vi "Init.vi"(5 "PathControl.lvclass":refnum<class "PathControl.lvclass">, 6 "Environmental classes":refnum<class "Instrument.lvclass">[](array[class]), 7 "XML Handler.lvclass":refnum<class "XML Handler.lvclass">, 8 "error in (no error)":errorcluster, 9 "Instruments to Use":T1(array[cluster]), 10 "Device.lvclass":refnum<class "Device.lvclass">, 11 "Power Meter GUI in":refnum<class "Power Meter GUI.lvclass">) -> (0 "error out":errorcluster, 3 "Power Meter GUI out":refnum<class "Power Meter GUI.lvclass">)   [LabVIEW 2020, in "Power Meter GUI.lvclass"]
doc: "Initializes the measurement.\nThis verifies that the instruments are present and adds them into the class data.\nIs also adds the xml handler into the class data."
uses:
  Power Meter GUI.lvclass
  C:/Sandbox/RF Bench/Source Code/WiSpry Test Framework/Measurements/Measurement.lvclass
  Devices/Device.lvclass
  Instruments/Instrument.lvclass
  XML Handler/XML Handler.lvclass
  Path Control/PathControl.lvclass
  Controls/Init State Machine.ctl
  Instruments/Power Meter/Power Meter.lvclass
  Measurement.lvclass/Measurement.ctl
  Measurement.lvclass
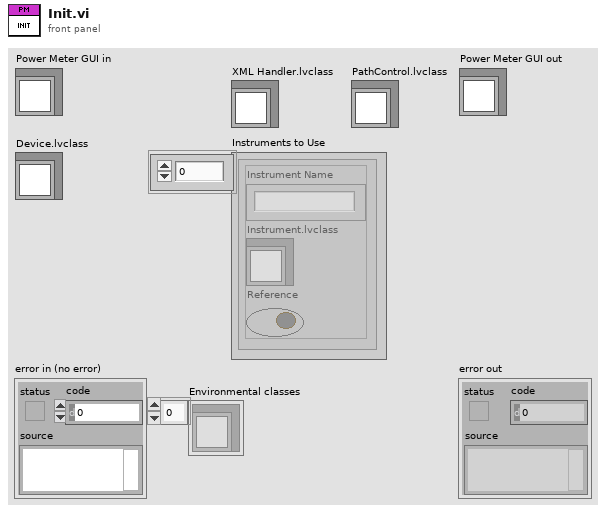
[diagram p1: front panel]
types:
  T1 = cluster{"Instrument Name":string, "Instrument.lvclass":refnum<class "Instrument.lvclass">, "Reference":bool}[]
  T2 = typedef "Power Meter GUI.lvclass/Init State Machine.ctl" = enum16{"Verify Instruments", "Init Instruments", "Init Device", "Create test in XML", "Set Path", "Done"}
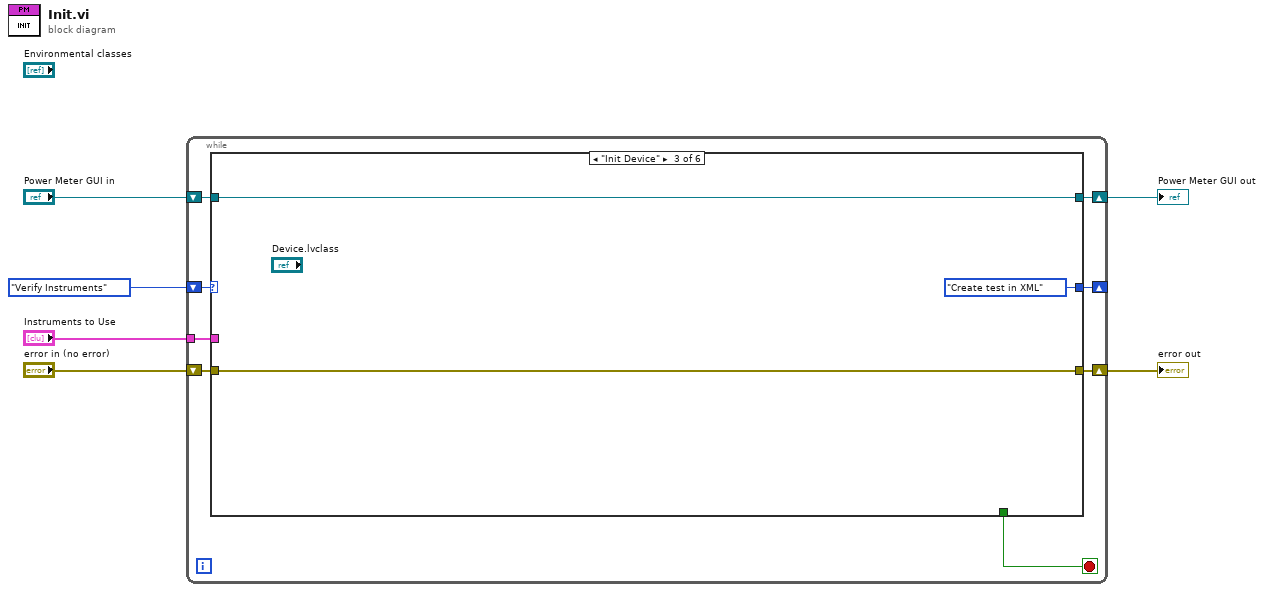
[diagram p0: block diagram]
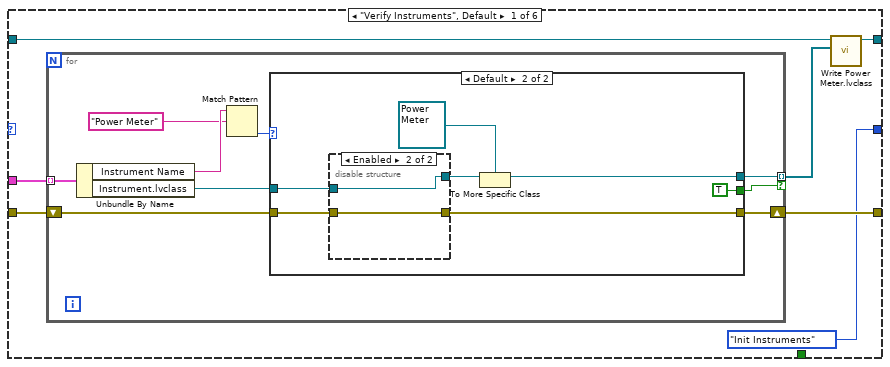
[diagram p2: hidden frame]
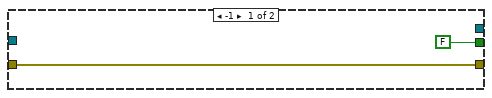
[diagram p3: hidden frame]
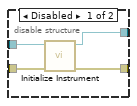
[diagram p4: hidden frame]
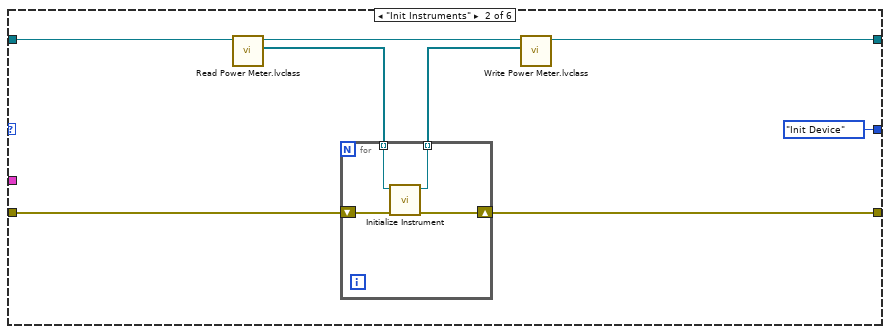
[diagram p5: hidden frame]
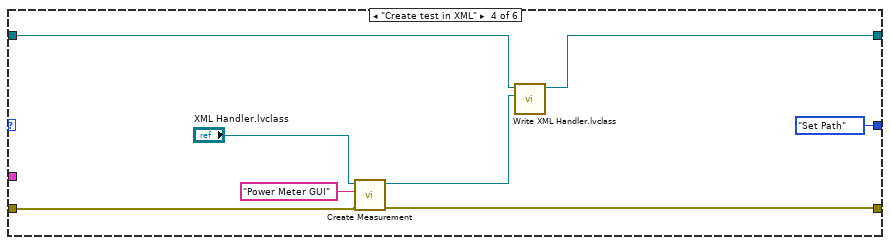
[diagram p6: hidden frame]
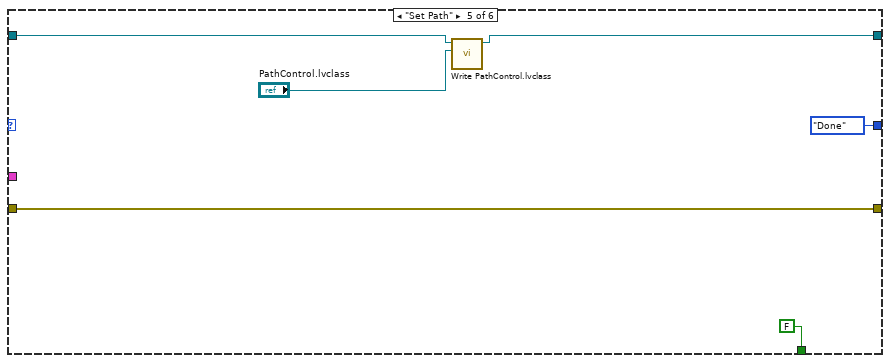
[diagram p7: hidden frame]
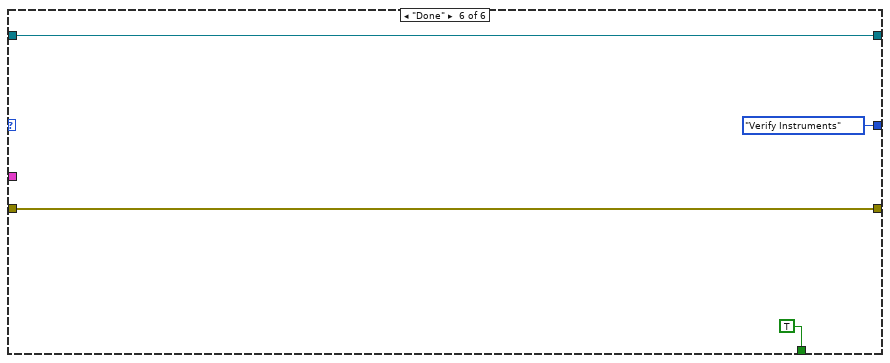
[diagram p8: hidden frame]
diagram:
  n1 = while {
    tunnel: "Instruments to Use" -> [w12]
    shift-right: [w14] -> w6
    shift-left: "error in (no error)" -> [w13]
    shift-right: [w10] -> w2
    shift-left: "Power Meter GUI in" -> [w11]
    shift-right: [w8] -> _
    shift-left: Init_State_Machine."Verify Instruments" ("States") -> [w9]
    stop <- w7 stop-if-true
    n2 = case shown="\"Init Device\"" w9 {
      tunnel: [w21 w51 w59 w64 w73 w77] -> w14
      tunnel: w13 -> [w20 w52 w59 w65 w73 w77]
      tunnel: w12 -> [w19 _ _ _ _ _]
      tunnel: w11 -> [w18 w48 w58 w62 w71 w75]
      tunnel: [w17 w46 w58 w63 w70 w75] -> w10
      tunnel: [Init_State_Machine."Init Instruments" ("States") Init_State_Machine."Init Device" ("States") Init_State_Machine."Create test in XML" ("States") Init_State_Machine."Set Path" ("States") Init_State_Machine."Done" ("States") Init_State_Machine."Verify Instruments" ("States")] -> w8
      tunnel: [_ _ _ _ FALSE TRUE] -> w7
      frame "Verify Instruments", Default {
        n3 = for {
          shift-right: [w29] -> w21
          shift-left: w20 -> [w30]
          tunnel: w19 -> [w28] mode=indexing
          tunnel: [w23] -> w16 mode=indexing if=w22
          n4 = Unbundle By Name(w28) -> ("Instrument Name"=w26:string, "Instrument.lvclass"=w27:refnum<class "Instrument.lvclass">)
          n5 = Match Pattern(string=w26, regular expression="Power Meter") -> (offset past match=w24:i32)  [unwired: 1 in, 3 out]
          n6 = case shown="Default" w24 {
            tunnel: w30 -> [w32 w39]
            tunnel: [w32 w34] -> w29
            tunnel: w27 -> [_ w36]
            tunnel: [_ w37] -> w23
            tunnel: [FALSE TRUE] -> w22
            frame -1 {
            }
            frame Default {
              n7 = disable-structure shown="Enabled" {
                disable-tunnel: w39 -> [w43 w45]
                disable-tunnel: w36 -> [w42 w44]
                disable-tunnel: [w41 w44] -> w35
                disable-tunnel: [w40 w45] -> w34
                frame Disabled {
                  n8 = call-dynamic "Initialize Instrument.vi"("error in (no error)"=w43, "Instrument in"=w42) -> ("error out"=w40:errorcluster, "Instrument out"=w41:refnum<class "Instrument.lvclass">)  [unwired: 8 in]
                }
                frame Enabled {
                }
              }
              n9 = To More Specific Class(target class=refnum<class "Power Meter.lvclass"> refnum ("Power Meter.lvclass"), reference=w35) -> (specific class reference=w37:refnum<class "Power Meter.lvclass">)  [unwired: 1 in, 1 out]
            }
          }
        }
        n10 = call-dynamic "Write Power Meter.lvclass.vi"("Power Meters"=w16, "Power Meter GUI in"=w18) -> ("Power Meter GUI out"=w17:refnum<class "Power Meter GUI.lvclass">)  [unwired: 9 in]
      }
      frame "Init Instruments" {
        n11 = call-dynamic "Read Power Meter.lvclass.vi"("Power Meter GUI in"=w48) -> ("Power Meters"=w50:refnum<class "Power Meter.lvclass">[], "Power Meter GUI out"=w47:refnum<class "Power Meter GUI.lvclass">)  [unwired: 9 in]
        n12 = for {
          shift-right: [w56] -> w51
          shift-left: w52 -> [w57]
          tunnel: w50 -> [w55] mode=indexing
          tunnel: [w54] -> w49 mode=indexing
          n13 = call-dynamic "Initialize Instrument.vi"("error in (no error)"=w57, "Instrument in"=w55) -> ("error out"=w56:errorcluster, "Instrument out"=w54:refnum<class "Power Meter.lvclass">)  [unwired: 8 in]
        }
        n14 = call-dynamic "Write Power Meter.lvclass.vi"("Power Meters"=w49, "Power Meter GUI in"=w47) -> ("Power Meter GUI out"=w46:refnum<class "Power Meter GUI.lvclass">)  [unwired: 9 in]
      }
      frame "Init Device" {
      }
      frame "Create test in XML" {
        n15 = call "Create Measurement.vi"("error in (no error)"=w65, "Measurement Name"="Power Meter GUI", "XML Handler in"="XML Handler.lvclass") -> ("error out"=w64:errorcluster, "XML Handler out"=w66:refnum<class "XML Handler.lvclass">)  [unwired: 7 in]
        n16 = call "Write XML Handler.lvclass.vi"("XML Handler.lvclass"=w66, "Measurements in"=w62) -> ("Measurements out"=w63:refnum<class "Power Meter GUI.lvclass">)  [unwired: 9 in]
      }
      frame "Set Path" {
        n17 = call "Write PathControl.lvclass.vi"("PathControl.lvclass"="PathControl.lvclass", "Measurements in"=w71) -> ("Measurements out"=w70:refnum<class "Power Meter GUI.lvclass">)  [unwired: 9 in]
      }
      frame "Done" {
      }
    }
  }
  "error out" <- w6
  "Power Meter GUI out" <- w2
